vi "TestPID.vi"() -> ()   [LabVIEW 2016]
uses:
  <vilib>/Rock Robotics/WPI/ThirdParty/CanMotor/TalonSRX/WPI_CANTalonSRX_APIControlMode.ctl
  <vilib>/Rock Robotics/WPI/ThirdParty/CanMotor/TalonSRX/WPI_CANTalonSRX_APIFeedbackSelect.ctl
panel:
  in  "D":dbl
  in  "I":dbl
  in  "P":dbl=16.0
  in  "a or b":bool=TRUE
  in  "b":dbl=200.0
  in  "a":dbl=900.0
  out "Waveform Chart":cluster{"Output":dbl, "Sensor Position":dbl}(graph)={"Output"=900.0, "Sensor Position"=902.0}
  in  "setpoint":dbl format="%.2f"
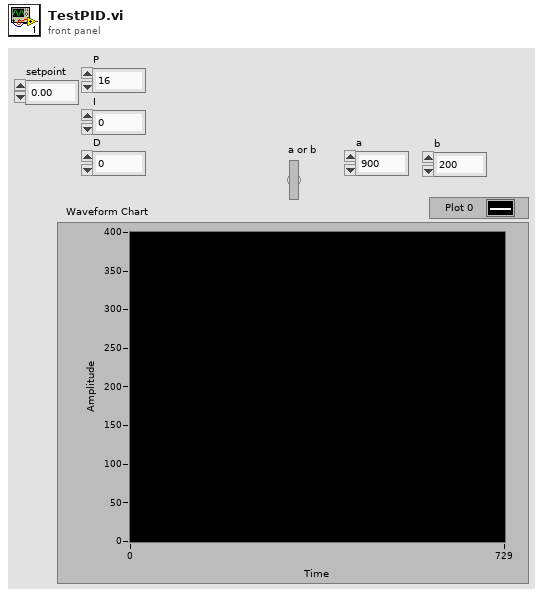
[diagram p1: front panel]
types:
  T1 = typedef "WPI_CANTalonSRX_APIFeedbackSelect.ctl" = enum16{"Digital Quadrature Encoder", "Analog Potentiometer", "Analog Encoder", "Count on Quad-A (Rising-Edge)", "Count on Quad-A (Falling-Edge)", "CTR Magnetic Enc (Absolute)", "CTR Magnetic Enc (Relative)", "Pulse Width"}
  T2 = typedef "WPI_CANTalonSRX_APIControlMode.ctl" = enum8{"Percent VBus", "Speed", "Position", "Slave", "Unchanged / Invalid", "Voltage Compensation", "Current", "Motion Profile", "Motion Magic"}
  T3 = typedef "WPI_MotorControlDeviceRef.ctl" = cluster{"DeviceStatus":errorcluster, "Type":T4, "PWM":cluster{"PWM Channel":T5, "DeadBand":T6}, "CAN":cluster{"Device Number":u8, "SetOutput VI Ref":variant, "GetOutput VI Ref":variant, "Enable VI Ref":variant, "Disable VI Ref":variant, "Data":variant}, "Invert":bool}
  T4 = typedef "WPI_MotorControlType.ctl" = enum16{"PWM", "CAN"}
  T5 = typedef "FPGA_DIOPWMChannel.ctl" = enum8{"PWM 0", "PWM 1", "PWM 2", "PWM 3", "PWM 4", "PWM 5", "PWM 6", "PWM 7", "PWM 8", "PWM 9", "PWM MXP 0", "PWM MXP 1", "PWM MXP 2", "PWM MXP 3", "PWM MXP 4", "PWM MXP 5", "PWM MXP 6", "PWM MXP 7", "PWM MXP 8", "PWM MXP 9", "Invalid"}
  T6 = typedef "WPI_PWMDeadband.ctl" = cluster{"Name":string, "maxPositivePwm":i32, "minPositivePwm":i32, "centerPwm":i32, "maxNegativePwm":i32, "minNegativePwm":i32, "angularRange":u16}
  T7 = typedef "WPI_CANTalonSRX_GlobalStatus.ctl" = cluster{"Applied Throttle":dbl, "Module Enabled":bool, "CAN Error":errorcluster, "Closed Loop Error":dbl, "Forward Limit Switch Closed":bool, "Reverse Limit Switch Closed":bool, "Sensor Position":dbl, "Sensor Velocity":dbl, "Current":dbl, "Sticky Fault - Over Temp":bool, "Sticky Fault - Under Voltage":bool, "Sticky Fault - Forward Limit":bool, "Sticky Fault - Reverse Limit":bool, "Sticky Fault - Forward Soft Limit":bool, "Sticky Fault - Reverse Soft Limit":bool, "Brake is Enabled":bool, "Encoder Position":dbl, "Encoder Velocity":dbl, "Encoder Index Count":dbl, "Encoder A Pin State":bool, "Encoder B Pin State":bool, "Encoder Index Pin State":bool, "Analog In":dbl, "Analog In Velocity":dbl, "Temperature (C)":dbl, "Battery Voltage":dbl, "Control 5 Is Supported":bool, "Current Profile Slot Select":dbl, "Pos Div 8":bool, "Vel Div 4":bool, "Pulse Width Position":i32, "Pulse Width Velocity":i32, "Pulse Width Rise To Rise (us)":i32, "Pulse Width Rise To Fall (us)":i32, "Mot Prof Active Is Under Run":bool, "Mot Prof Active Has Under Run":bool, "Mot Prof Active Is Last":bool, "Mot Prof Active Velocity Only":bool, "Mot Prof Active Is Valid":bool, "Mot Prof Buffer Is Full":bool, "Mot Prof Active Profile Slot Select":i32, "Mot Prof NextID":i32, "Mot Prof Count":i32, "Mot Prof Active Velocity":dbl, "Mot Prof Active Position":dbl, "Mot Prof Output Enable":i32, "UsageFrame":u32, "Motion Magic Active Trajectory":cluster{"Velocity":dbl, "Position":dbl}}
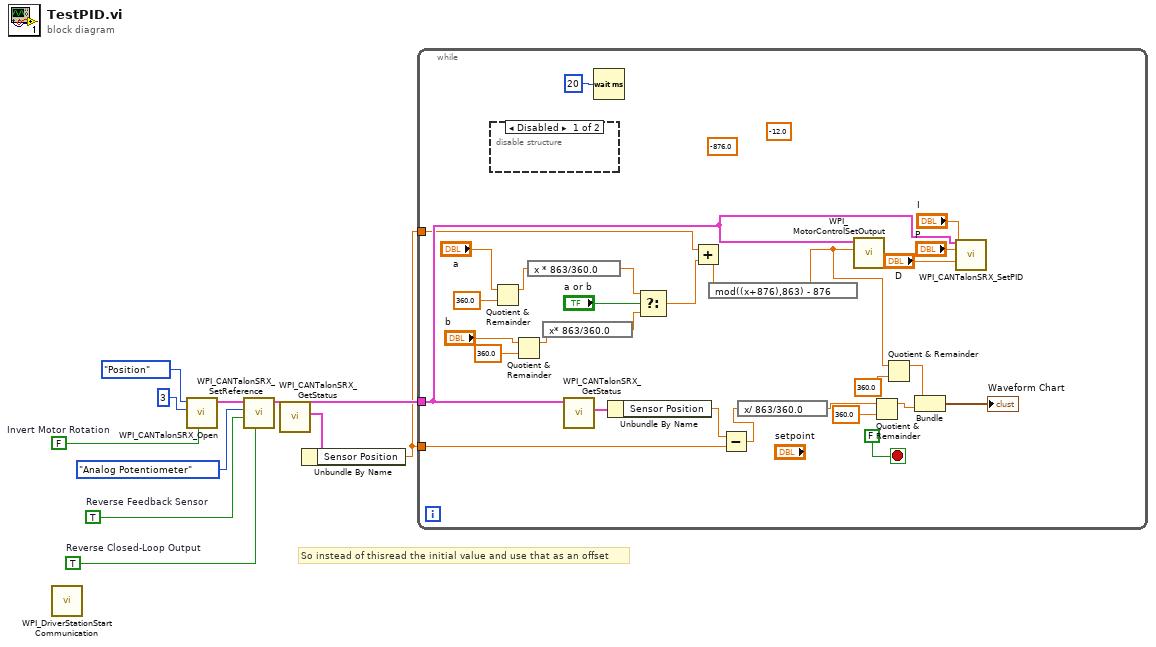
[diagram p0: block diagram]
diagram:
  w5 = FALSE  # Invert Motor Rotation
  w6 = TRUE  # Reverse Closed-Loop Output
  w7 = TRUE  # Reverse Feedback Sensor
  # "So instead of thisread the initial value and use that as an offset"
  n1 = call <vilib>:"WPI_DriverStationStart Communication.vi"() -> ()  [unwired: 12 in]
  n2 = call <vilib>:"WPI_CANTalonSRX_Open.vi"("Invert"=w5, "Device Number"=u8 3, "Control Mode"=WPI_CANTalonSRX_APIControlMode."Position") -> ("CAN Talon SRX Ref"=w8:T3)  [unwired: 7 in, 1 out]
  n3 = call <vilib>:"WPI_CANTalonSRX_SetReference.vi"("Reverse Closed-Loop Output"=w6, "Reverse Feedback Sensor"=w7, "Feedback Reference"=WPI_CANTalonSRX_APIFeedbackSelect."Analog Potentiometer", "CAN Talon SRX Ref"=w8) -> ("CAN Talon SRX Ref"=w4:T3)  [unwired: 6 in, 1 out]
  n4 = call <vilib>:"WPI_CANTalonSRX_GetStatus.vi"("CAN Talon SRX Ref"=w4) -> ("Talon SRX Status"=w2:T7, "CAN Talon SRX Ref"=w3:T3)  [unwired: 8 in, 1 out]
  n5 = Unbundle By Name(w2) -> ("Sensor Position"=w1:dbl)
  n6 = while {
    tunnel: w3 -> [w33]
    tunnel: w1 -> [w26]
    tunnel: w1 -> [w24]
    stop <- FALSE stop-if-true
    (unwired) -12.0 ("lower limit")
    (unwired) -876.0 ("upper limit")
    n7 = disable-structure shown="Disabled" {
      frame Disabled {
      }
      frame Enabled {
      }
    }
    n8 = Quotient & Remainder(x="a", y=360.0) -> (x-y*floor(x/y)=w16:dbl)  [unwired: 1 out]
    n9 = Quotient & Remainder(x="b", y=360.0) -> (x-y*floor(x/y)=w13:dbl)  [unwired: 1 out]
    n10 = expression code="x * 863/360.0"(w16) -> (w20:dbl)
    n11 = expression code="x* 863/360.0"(w13) -> (w19:dbl)
    n12 = call <vilib>:"WPI_CANTalonSRX_GetStatus.vi"("CAN Talon SRX Ref"=w33) -> ("Talon SRX Status"=w38:T7)  [unwired: 8 in, 2 out]
    n13 = Wait (ms)(milliseconds to wait=u32 20) -> ()  [unwired: 1 out]
    n14 = Unbundle By Name(w38) -> ("Sensor Position"=w25:dbl)
    n15 = Select(t=w20, s="a or b", f=w19) -> (s? t:f=w22:dbl)
    n16 = Add(x=w26, y=w22) -> (x+y=w21:dbl)
    n17 = expression code="mod((x+876),863) - 876"(w21) -> (w12:dbl)
    n18 = Subtract(x=w25, y=w24) -> (x-y=w23:dbl)
    n19 = expression code="x/ 863/360.0"(w23) -> (w31:dbl)
    n20 = call <vilib>:"WPI_MotorControlSetOutput.vi"("Output"=w12, "MotorControlDevRef"=w33) -> ()  [unwired: 7 in, 3 out]
    n21 = Quotient & Remainder(x=w31, y=360.0) -> (x-y*floor(x/y)=w27:dbl)  [unwired: 1 out]
    n22 = Quotient & Remainder(x=w12, y=360.0) -> (x-y*floor(x/y)=w28:dbl)  [unwired: 1 out]
    n23 = Bundle(w28, w27) -> (→"Waveform Chart":cluster{dbl, dbl})  [unwired: 1 in]
    n24 = call <vilib>:"WPI_CANTalonSRX_SetPID.vi"("CAN Talon SRX Ref"=w33, "P"="P", "I"="I", "D"="D") -> ()  [unwired: 10 in, 2 out]
  }
